vi "Engine Status.vi"(8 "error in (no error)":errorcluster, 11 "bt_System in":refnum<class "bt_System.lvclass">) -> (0 "error out":errorcluster, 2 "Idle?":bool, 3 "bt_System out":refnum<class "bt_System.lvclass">)   [LabVIEW 2021, in "BT.lvlib" / "bt_System.lvclass"]
uses:
  bt_System.lvclass
  bt_System.lvclass/bt_System.ctl
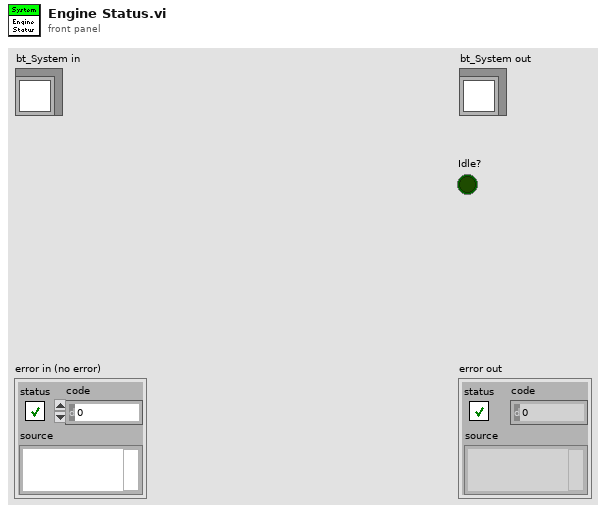
[diagram p1: front panel]
types:
  T1 = enum32{"Bad", "Idle", "Run top level", "Running"}
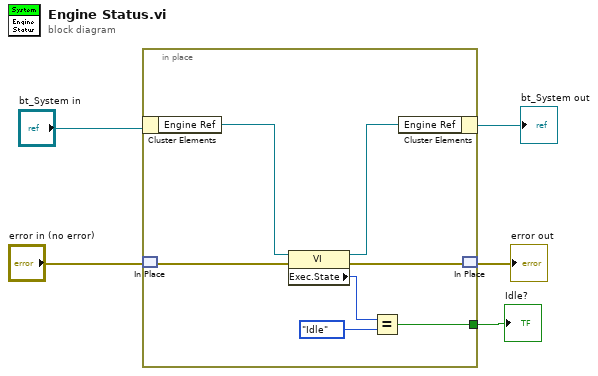
[diagram p0: block diagram]
diagram:
  n1 = in-place {
    in-place-border: [w6] -> w1
    n2 = in-place-cluster #1("bt_System in") -> ("Engine Ref"=w12:refnum<vi>)
    n3 = in-place-match #2("error in (no error)") -> (w9:errorcluster)
    n4 = property class="VI"(reference=w12, error in=w9) -> (reference out=w7:refnum<vi>, error out=w8:errorcluster, "Exec.State"=w11:T1)
    n5 = Equal?(x=w11, y=T1."Idle") -> (x = y?=w6:bool)
    n6 = in-place-cluster #1("Engine Ref"=w7) -> (→"bt_System out":refnum<class "bt_System.lvclass">)
    n7 = in-place-match #2(w8) -> (→"error out":errorcluster)
  }
  "Idle?" <- w1
